vi "CtrlEvents.vi"() -> ()   [LabVIEW 2014]
uses:
  <vilib>/event_ctls.llb/lveventtype.ctl
panel:
  out "String":string="Null,Timeout,Annotation Menu Selection,Annotation Menu Selection?,App Instance Close,App Instance Close?,Autoscale Range Change,Bookmark Info Change,Cell Edit,Cell Edit?,Cursor Grab,Cursor Grab?,Cursor Menu Selection,Cursor Menu Selection?,Cursor Move,Cursor Release,Data Change,Direction Change,Display State Change,Drag Ended,Drag Enter,Drag Leave,Drag Over,Drag Source Update,Drag Starting,Drag Starting?,Drop,Exec State Change,Key Down,Key Down?,Key Repeat,Key Repeat?,Key Up,Listbox Double Click,Menu Activation?,Menu Selection (App),Menu Selection? (App),Menu Selection (User),Mouse Down,Mouse Down?,Mouse Enter,Mouse Leave,Mouse Move,Mouse Up,Mouse Wheel,NI Security User Change (App),Pane Size,Panel Close,Panel Close?,Panel Resize,Plot Attribute Change,Scale Range Change,Shortcut Menu Activation?,Shortcut Menu Selection (App),Shortcut Menu Selection? (App),Shortcut Menu Selection (User),Tree Double Click,Tree Drag,Tree Drag?,Tree Drop,Tree Drop?,Tree Item Close,Tree Item Close?,Tree Item Open,Tree Item Open?,User Event,Value Change,Null,Timeout,Annotation Menu Selection,Annotation Menu Selection?,App Instance Close,App Instance Close?,Autoscale Range Change,Bookmark Info Change,Cell Edit,Cell Edit?,Cursor Grab,Cursor Grab?,Cursor Menu Selection,Cursor Menu Selection?,Cursor Move,Cursor Release,Data Change,Direction Change,Display State Change,Drag Ended,Drag Enter,Drag Leave,Drag Over,Drag Source Update,Drag Starting,Drag Starting?,Drop,Exec State Change,Key Down,Key Down?,Key Repeat,Key Repeat?,Key Up,Listbox Double Click,Menu Activation?,Menu Selection (App),Menu Selection? (App),Menu Selection (User),Mouse Down,Mouse Down?,Mouse Enter,Mouse Leave,Mouse Move,Mouse Up,Mouse Wheel,NI Security User Change (App),Pane Size,Panel Close,Panel Close?,Panel Resize,Plot Attribute Change,Scale Range Change,Shortcut Menu Activation?,Shortcut Menu Selection (App),Shortcut Menu Selection? (App),Shortcut Menu Selection (User),Tree Double Click,Tree Drag,Tree Drag?,Tree Drop,Tree Drop?,Tree Item Close,Tree Item Close?,Tree Item Open,Tree Item Open?,User Event,Value Change,"
  in  "Type":T1=enum."Value Change"
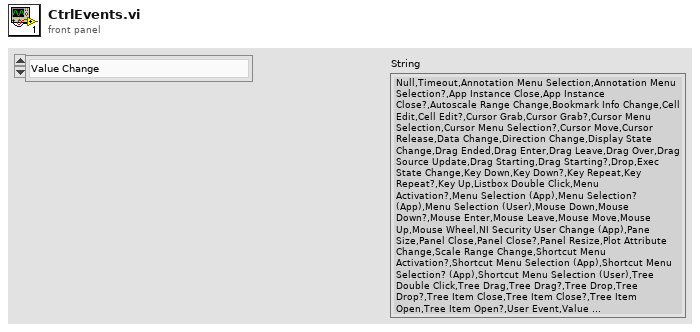
[diagram p1: front panel]
types:
  T1 = typedef "lveventtype.ctl" = enum32{"Null", "Timeout", "Annotation Menu Selection", "Annotation Menu Selection?", "App Instance Close", "App Instance Close?", "Autoscale Range Change", "Bookmark Info Change", "Cell Edit", "Cell Edit?", "Cursor Grab", "Cursor Grab?", "Cursor Menu Selection", "Cursor Menu Selection?", "Cursor Move", "Cursor Release", "Data Change", "Direction Change", "Display State Change", "Drag Ended", "Drag Enter", "Drag Leave", "Drag Over", "Drag Source Update", "Drag Starting", "Drag Starting?", "Drop", "Exec State Change", "Key Down", "Key Down?", "Key Repeat", "Key Repeat?", "Key Up", "Listbox Double Click", "Menu Activation?", "Menu Selection (App)", "Menu Selection? (App)", "Menu Selection (User)", "Mouse Down", "Mouse Down?", "Mouse Enter", "Mouse Leave", "Mouse Move", "Mouse Up", "Mouse Wheel", "NI Security User Change (App)", "Pane Size", "Panel Close", "Panel Close?", "Panel Resize", "Plot Attribute Change", "Scale Range Change", "Shortcut Menu Activation?", "Shortcut Menu Selection (App)", "Shortcut Menu Selection? (App)", "Shortcut Menu Selection (User)", "Tree Double Click", "Tree Drag", "Tree Drag?", "Tree Drop", "Tree Drop?", "Tree Item Close", "Tree Item Close?", "Tree Item Open", "Tree Item Open?", "User Event", "Value Change"}
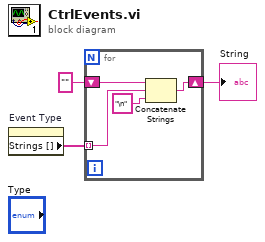
[diagram p0: block diagram]
diagram:
  n1 = property on="Event Type" class="Enum (strict)"() -> ("Strings []"=w3:string[])  [unwired: 2 in, 2 out]
  n2 = for {
    tunnel: w3 -> [w7] mode=indexing
    shift-right: [w6] -> w2
    shift-left: "" -> [w5]
    n3 = Concatenate Strings(w5, w7, "\n" ("string")) -> (w6:string)
  }
  "String" <- w2
